vi "Update Channel Parameters.vi"(7 "Digital":bool=TRUE, 8 "error in (no error)":errorcluster, 9 "Sequence Number":i32, 10 "Number of Channels":i32, 11 "Plugin in":refnum<class "Sequencer with Output Values.lvclass">) -> (0 "error out":errorcluster, 1 "Names":string[](array[string]), 2 "Values":string[](array[string]), 3 "Plugin out":refnum<class "Sequencer with Output Values.lvclass">)   [LabVIEW 2024, in "Sequencer with Output Values.lvlib" / "Sequencer with Output Values.lvclass"]
uses:
  Sequencer with Output Values.lvclass
  C:/Program Files/National Instruments/LabVIEW 2024/vi.lib/FlexLogger/SDK/PluginSDK.lvlibp/PEFClasses/SDK/Plugin/Plugin.lvclass
  Global Strings.vi
  <vilib>/FlexLogger/SDK/PluginSDK.lvlibp/PEFClasses/SDK/Plugin/ParameterAccess/Read String.vi
  <vilib>/FlexLogger/SDK/PluginSDK.lvlibp/PEFClasses/SDK/Plugin/ParameterAccess/Write String.vi
  <vilib>/FlexLogger/SDK/PluginSDK.lvlibp/PEFClasses/SDK/Plugin/Plugin.lvclass
  C:/Program Files/National Instruments/LabVIEW 2024/vi.lib/FlexLogger/SDK/PluginSDK.lvlibp/PEFClasses/SDK/Processing Element/Processing Element.lvclass
  C:/dev/niflexlogger-plugins/plugins/Sequencer with Output Values/source/Sequencer with Output Values/Sequencer with Output Values.lvclass
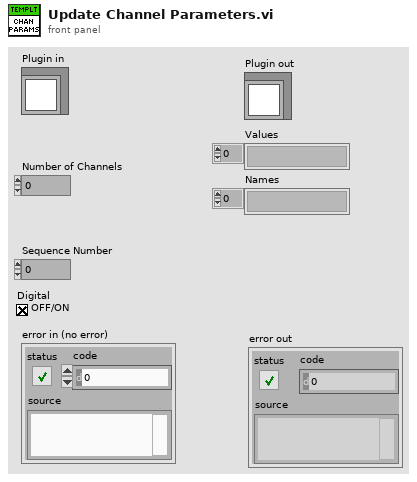
[diagram p1: front panel]
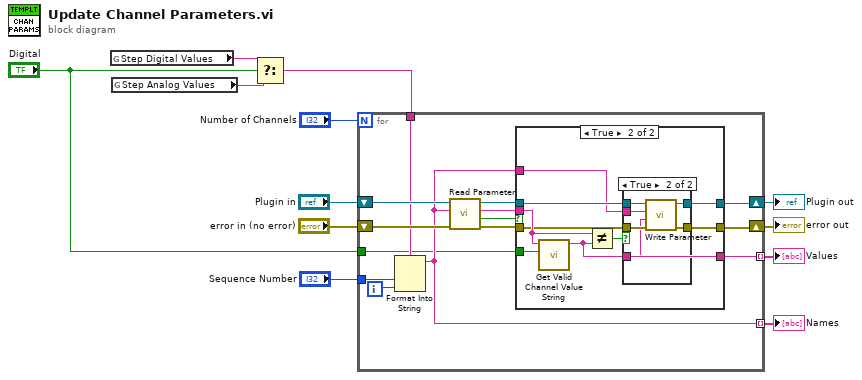
[diagram p0: block diagram]
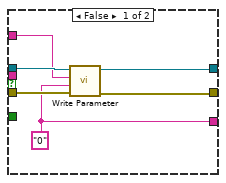
[diagram p2: hidden frame]
diagram:
  n1 = global read "Global Strings.vi" "Step Digital Values"() -> (w4:string)
  n2 = global read "Global Strings.vi" "Step Analog Values"() -> (w3:string)
  n3 = Select(t=w4, s="Digital", f=w3) -> (s? t:f=w2:string)
  n4 = for {
    N: "Number of Channels" -> [_]
    tunnel: "Sequence Number" -> [w26]
    shift-right: [w16] -> w6
    shift-left: "Plugin in" -> [w24]
    shift-right: [w15] -> w5
    shift-left: "error in (no error)" -> [w23]
    tunnel: w2 -> [w22]
    tunnel: [w18] -> w7 mode=indexing
    tunnel: [w14] -> w8 mode=indexing
    tunnel: "Digital" -> [w13]
    i -> [w25]
    n5 = Format Into String(format string=w22, w26, w25) -> (resulting string=w18:string)  [unwired: 2 in, 1 out]
    n6 = call-poly <vilib>:"Read Parameter.vi"("error in (no error)"=w23, "Name"=w18, "Plugin in"=w24) -> ("error out"=w17:errorcluster, "Found"=w21:bool, "Value"=w19:string, "Plugin out"=w20:refnum<class "Sequencer with Output Values.lvclass">)  [unwired: 5 in]
    n7 = case shown="True" w21 {
      tunnel: w20 -> [w32 w38]
      tunnel: w17 -> [w31 w37]
      tunnel: [w30 w36] -> w16
      tunnel: [w29 w35] -> w15
      tunnel: w18 -> [w28 w34]
      tunnel: w19 -> [_ w40]
      tunnel: [w27 w33] -> w14
      tunnel: w13 -> [_ w41]
      frame False {
        w27 = "0"
        n8 = call-poly <vilib>:"Write Parameter.vi"("error in (no error)"=w31, "Value"=w27, "Name"=w28, "Plugin in"=w32) -> ("error out"=w29:errorcluster, "Plugin out"=w30:refnum<class "Sequencer with Output Values.lvclass">)  [unwired: 6 in]
      }
      frame True {
        n9 = call "Get Valid Channel Value String.vi"("Digital"=w41, "Channel Values"=w40) -> ("Valid Channel Values"=w33:string)  [unwired: 9 in]
        n10 = Not Equal?(x=w40, y=w33) -> (x != y?=w39:bool)
        n11 = case shown="True" w39 {
          tunnel: w38 -> [w43 w49]
          tunnel: w37 -> [w42 w48]
          tunnel: [w43 w47] -> w36
          tunnel: [w42 w46] -> w35
          tunnel: w34 -> [_ w45]
          tunnel: w33 -> [_ w44]
          frame False {
          }
          frame True {
            n12 = call-poly <vilib>:"Write Parameter.vi"("error in (no error)"=w48, "Value"=w44, "Name"=w45, "Plugin in"=w49) -> ("error out"=w46:errorcluster, "Plugin out"=w47:refnum<class "Sequencer with Output Values.lvclass">)  [unwired: 6 in]
          }
        }
      }
    }
  }
  "Values" <- w8
  "Names" <- w7
  "Plugin out" <- w6
  "error out" <- w5
